vi "FormatDMAelement_2.vi"(8 "valid in":bool, 9 "c(t) - AM":fxp<+/-,32,21>, 10 "c(t) - Phase":fxp<+/-,32,4>, 11 "Data in":fxp<+/-,16,14>[](array[numeric])=[0.0, 0.0, 0.0, 0.0]) -> (0 "valid out":bool, 3 "Element":u64[](array[numeric]))   [LabVIEW 2013]
uses:
  <vilib>/rvi/FXPMathLib/FxpInterpret/XNode/nifxpmath_Interpret.xnode
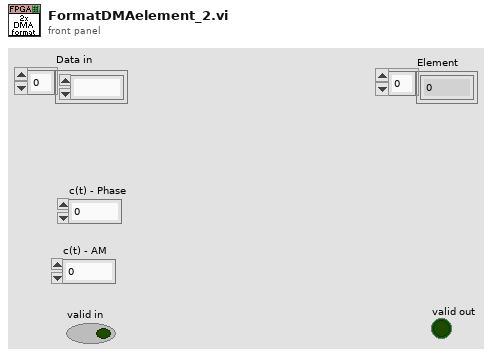
[diagram p1: front panel]
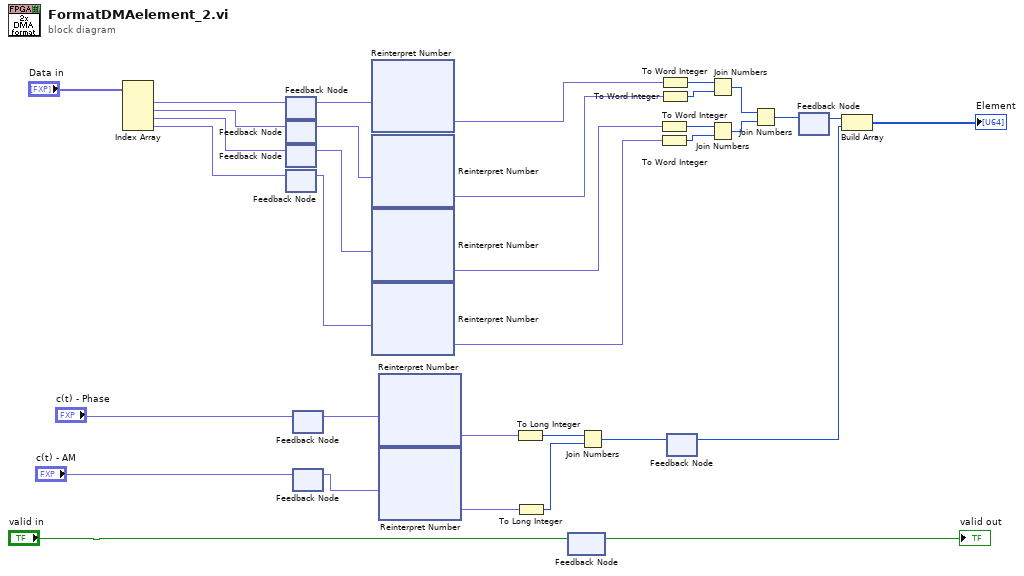
[diagram p0: block diagram]
diagram:
  n1 = Index Array(array="Data in") -> (element #1=w30:fxp<+/-,16,14>, element #2=w29:fxp<+/-,16,14>, element #3=w28:fxp<+/-,16,14>, element #4=w27:fxp<+/-,16,14>)  [unwired: 4 in]
  n2 = feedback #1() -> (w20:fxp<+/-,16,14>)  [unwired: 1 in]
  n3 = feedback-in #1(w30) -> ()
  n4 = feedback #2() -> (w18:fxp<+/-,16,14>)  [unwired: 1 in]
  n5 = feedback-in #2(w29) -> ()
  n6 = feedback #3() -> (w17:fxp<+/-,16,14>)  [unwired: 1 in]
  n7 = feedback-in #3(w28) -> ()
  n8 = feedback #4() -> (w16:fxp<+/-,16,14>)  [unwired: 1 in]
  n9 = feedback-in #4(w27) -> ()
  n10 = feedback #5() -> (w12:fxp<+/-,32,4>)  [unwired: 1 in]
  n11 = feedback-in #5("c(t) - Phase") -> ()
  n12 = feedback #6() -> (w11:fxp<+/-,32,21>)  [unwired: 1 in]
  n13 = feedback-in #6("c(t) - AM") -> ()
  n14 = xnode "Reinterpret Number"("x"=w20) -> ("y"=w19:fxp<+/-,16,16>)
  n15 = xnode "Reinterpret Number"("x"=w18) -> ("y"=w15:fxp<+/-,16,16>)
  n16 = xnode "Reinterpret Number"("x"=w17) -> ("y"=w14:fxp<+/-,16,16>)
  n17 = xnode "Reinterpret Number"("x"=w16) -> ("y"=w13:fxp<+/-,16,16>)
  n18 = xnode "Reinterpret Number"("x"=w12) -> ("y"=w10:fxp<+/-,32,32>)
  n19 = xnode "Reinterpret Number"("x"=w11) -> ("y"=w9:fxp<+/-,32,32>)
  n20 = To Long Integer(number=w10) -> (32bit integer=w8:i32)
  n21 = To Long Integer(number=w9) -> (32bit integer=w7:i32)
  n22 = feedback #7() -> (→"valid out":bool)  [unwired: 1 in]
  n23 = feedback-in #7("valid in") -> ()
  n24 = Join Numbers(hi=w8, lo=w7) -> ((hi.lo)=w4:u64)
  n25 = To Word Integer(number=w14) -> (16bit integer=w24:i16)
  n26 = To Word Integer(number=w13) -> (16bit integer=w23:i16)
  n27 = To Word Integer(number=w19) -> (16bit integer=w25:i16)
  n28 = To Word Integer(number=w15) -> (16bit integer=w26:i16)
  n29 = feedback #8() -> (w3:u64)  [unwired: 1 in]
  n30 = feedback-in #8(w4) -> ()
  n31 = Join Numbers(hi=w25, lo=w26) -> ((hi.lo)=w22:u32)
  n32 = Join Numbers(hi=w24, lo=w23) -> ((hi.lo)=w21:u32)
  n33 = Join Numbers(hi=w22, lo=w21) -> ((hi.lo)=w6:u64)
  n34 = feedback #9() -> (w5:u64)  [unwired: 1 in]
  n35 = feedback-in #9(w6) -> ()
  n36 = Build Array(w5, w3) -> (→"Element":u64[])
